vi "runTypeToObject.vi"(11 "Run Type":T1(ring)) -> (2 "Alignment":u16(ring)=1 items=["LEFT"=1, "CENTER"=2, "RIGHT"=3, "BOTH"=4, "MEDIUM_KASHIDA"=5, "DISTRIBUTE"=6, "NUM_TAB"=7, "HIGH_KASHIDA"=8, "LOW_KASHIDA"=9, "THAI_DISTRIBUTE"=10], 3 "Run Type Object":refnum<class "xwpfRun.lvclass">)   [LabVIEW 2017, in "Word_Specific.lvlib" / "xwpfParagraph.lvclass"]
uses:
  xwpfParagraph.lvclass
  xwpfRun/xwpfRun.lvclass
  xwpfRun.Title/xwpfRun.Title.lvclass
  C:/Users/Neo/Desktop/Dev_Tools_BR/LabVIEW_NPOI/src/LabVIEW NPOI/xwpfRun/xwpfRun.lvclass
  xwpfRun.Header1/xwpfRun.Header1.lvclass
  xwpfRun.Header2/xwpfRun.Header2.lvclass
  xwpfRun.Header3/xwpfRun.Header3.lvclass
  xwpfRun.Normal/xwpfRun.Normal.lvclass
  xwpfRun.Figure/xwpfRun.Figure.lvclass
  xwpfRun.PageBreak/xwpfRun.PageBreak.lvclass
  xwpfRun/Get Alignement.vi
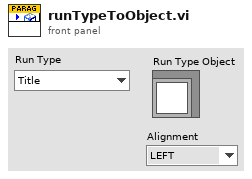
[diagram p1: front panel]
types:
  T1 = enum16{"Title", "Heading 1", "Heading 2", "Heading 3", "Normal", "Figure", "Page Break"}
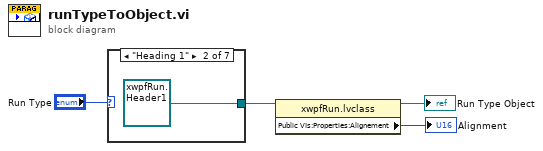
[diagram p0: block diagram]
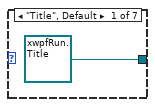
[diagram p2: hidden frame]
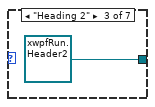
[diagram p3: hidden frame]
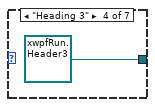
[diagram p4: hidden frame]
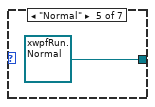
[diagram p5: hidden frame]
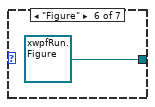
[diagram p6: hidden frame]
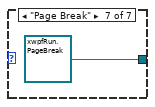
[diagram p7: hidden frame]
diagram:
  n1 = case shown="\"Heading 1\"" "Run Type" {
    tunnel: [refnum<class "xwpfRun.Title.lvclass"> refnum ("LabVIEW NPOI.lvlib:xwpfRun.Title.lvclass") refnum<class "xwpfRun.Header1.lvclass"> refnum ("LabVIEW NPOI.lvlib:xwpfRun.Header1.lvclass") refnum<class "xwpfRun.Header2.lvclass"> refnum ("LabVIEW NPOI.lvlib:xwpfRun.Header2.lvclass") refnum<class "xwpfRun.Header3.lvclass"> refnum ("LabVIEW NPOI.lvlib:xwpfRun.Header3.lvclass") refnum<class "xwpfRun.Normal.lvclass"> refnum ("LabVIEW NPOI.lvlib:xwpfRun.Normal.lvclass") refnum<class "xwpfRun.Figure.lvclass"> refnum ("LabVIEW NPOI.lvlib:xwpfRun.Figure.lvclass") refnum<class "xwpfRun.PageBreak.lvclass"> refnum ("LabVIEW NPOI.lvlib:xwpfRun.PageBreak.lvclass")] -> w3
    frame "Title", Default {
    }
    frame "Heading 1" {
    }
    frame "Heading 2" {
    }
    frame "Heading 3" {
    }
    frame "Normal" {
    }
    frame "Figure" {
    }
    frame "Page Break" {
    }
  }
  n2 = property class="xwpfRun.lvclass"(reference=w3) -> (reference out=→"Run Type Object":refnum<class "xwpfRun.lvclass">, "Public VIs:Properties:Alignement"=→"Alignment":u16)  [unwired: 1 in, 1 out]
